vi "setForceSetpointToForceMeasured.vi"(8 "error in (no error)":errorcluster, 11 "Model in":refnum<class "Model.lvclass">) -> (0 "error out":errorcluster, 3 "Model out":refnum<class "Model.lvclass">)   [LabVIEW 2013, in "Model.lvclass"]
uses:
  Model.lvclass
  Model.lvclass/Model.ctl
  ApplicationElements/ForceSensor/ForceSensor.lvclass/ForceSensor.ctl
  ApplicationElements/SystemController/SystemController.lvclass/SystemController.ctl
  ApplicationElements/ForceSensor/ForceSensor.lvclass
  ApplicationElements/SystemController/SystemController.lvclass
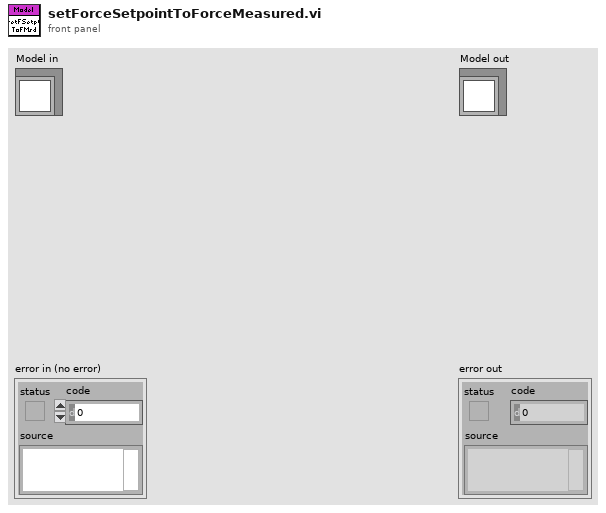
[diagram p1: front panel]
types:
  T1 = typedef "ForceDemand.ctl" = dbl[unit]
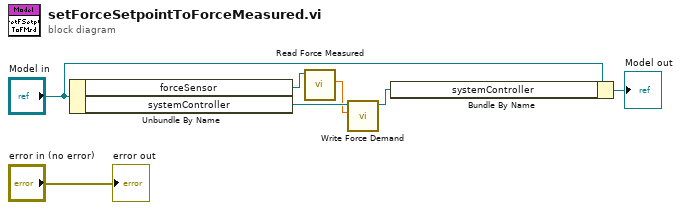
[diagram p0: block diagram]
diagram:
  n1 = Unbundle By Name("Model in") -> ("forceSensor"=w4:refnum<class "ForceSensor.lvclass">, "systemController"=w3:refnum<class "SystemController.lvclass">)
  n2 = call "Read Force Measured.vi"("ForceSensor in"=w4) -> ("Force Demand"=w2:T1)  [unwired: 9 in, 1 out]
  n3 = call "Write Force Demand.vi"("Force Demand"=w2, "SystemController in"=w3) -> ("SystemController out"=w1:refnum<class "SystemController.lvclass">)  [unwired: 9 in]
  n4 = Bundle By Name(cluster="Model in", "systemController"=w1) -> (→"Model out":refnum<class "Model.lvclass">)
  "error out" <- "error in (no error)"
